vi "Add Float SCTL 40 MHz Latency 0 Pipeline 0.vi"(1 "y":sgl, 2 "x":sgl) -> (0 "x+y":sgl)   [LabVIEW 2015]
uses:
  <vilib>/rvi/IPIntegrationNode/IPINode_Typedef/niFpgaIPINodeSupportedFamilies.ctl
  <vilib>/rvi/IPIntegrationNode/IPINode_Utilities/niFpgaIPINodeSimCore.vi
  <vilib>/rvi/XilinxIP/XIPIN_XNode/niFpgaXIPIN.xnode
  Add SCTL L0/Add_SCTL_L0_C3ADE5BE76064AA39E7EE6565DE88692.dll
  <vilib>/rvi/IPIntegrationNode/IPINode_Xnode/niFpgaIPINode.xnode
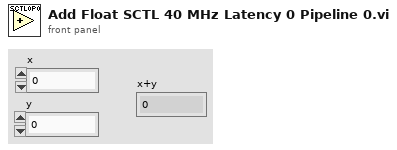
[diagram p1: front panel]
types:
  T1 = typedef "niFpgaIPINodeSupportedFamilies.ctl" = cluster{"unlimited?":bool, "supported targets":string[]}
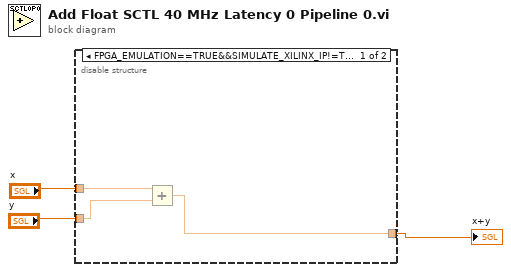
[diagram p0: block diagram]
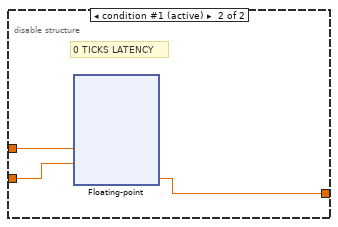
[diagram p2: hidden frame]
diagram:
  n1 = disable-structure shown="FPGA_EMULATION==TRUE&&SIMULATE_XILINX_IP!=TRUE, Default" {
    disable-tunnel: "x" -> [w6 w9]
    disable-tunnel: "y" -> [w5 w8]
    disable-tunnel: [w4 w7] -> w1
    frame condition #0 {
      n2 = Add(x=w6, y=w5) -> (x+y=w4:sgl)
    }
    frame condition #1 (active) {
      # "0 TICKS LATENCY"
      n3 = xnode ("Floating-point")("a"=w9, "b"=w8) -> ("result"=w7:sgl)
    }
  }
  "x+y" <- w1
